vi "showFrontEnd.vi"(8 "error in (no error)":errorcluster, 11 "StaticOutputEditor in":refnum<class "StaticOutputEditor.lvclass">) -> (0 "error out":errorcluster, 3 "StaticOutputEditor out":refnum<class "StaticOutputEditor.lvclass">)   [LabVIEW 2011, in "Views.lvlib" / "ScriptEditor.lvlib" / "StaticOutputEditor.lvclass"]
uses:
  StaticOutputEditor.lvclass
  StaticOutputEditor.lvclass/StaticOutputEditor.ctl
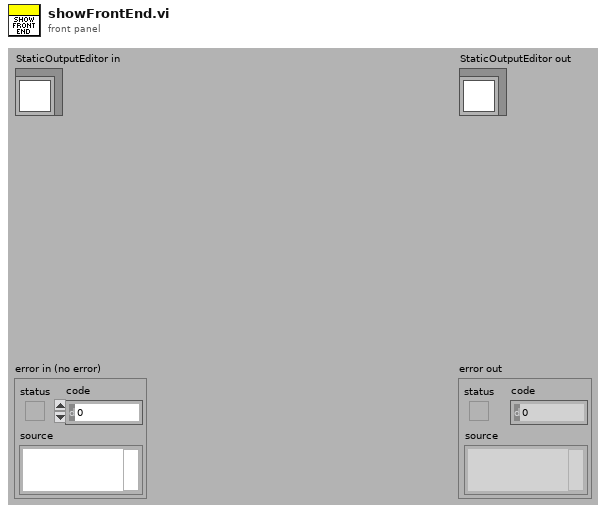
[diagram p1: front panel]
types:
  T1 = enum32{"Invalid", "Standard", "Closed", "Hidden", "Minimized", "Maximized"}
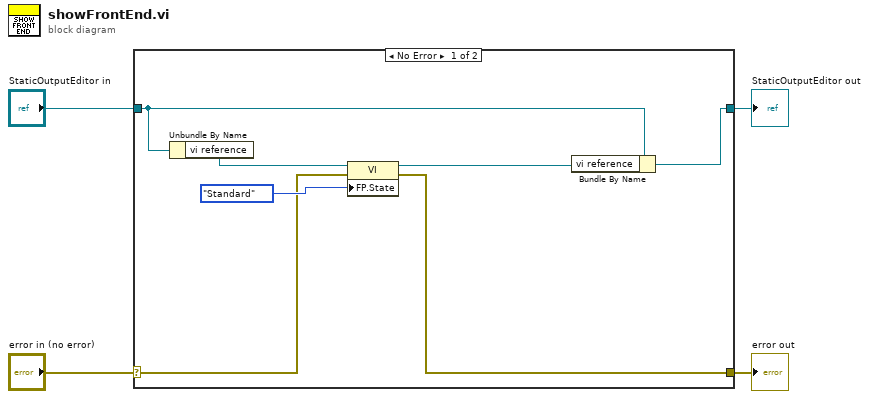
[diagram p0: block diagram]
diagram:
  n1 = case shown="No Error" "error in (no error)" {
    selector: "error in (no error)" -> [w9 w13]
    tunnel: [w8 w13] -> w3
    tunnel: [w6 w12] -> w1
    tunnel: "StaticOutputEditor in" -> [w7 w12]
    frame No Error {
      n2 = Unbundle By Name(w7) -> ("vi reference"=w11:refnum<vi>)
      n3 = property class="VI"(reference=w11, error in=w9, "FP.State"=T1."Standard" ("Front Panel Window:State")) -> (reference out=w5:refnum<vi>, error out=w8:errorcluster)
      n4 = Bundle By Name(cluster=w7, "vi reference"=w5) -> (w6:refnum<class "StaticOutputEditor.lvclass">)
    }
    frame Error {
    }
  }
  "error out" <- w3
  "StaticOutputEditor out" <- w1
